vi "Compass Loop.vi"   [LabVIEW 2009]
uses:
  <vilib>/Platform/TimedLoop/XDataNode/XDataNode.xnode
  <vilib>/Platform/TimedLoop/XDataNode/loadlvalarms.vi
  <vilib>/Platform/TimedLoop/XDataNode/timing_clust.ctl
  <vilib>/Platform/TimedLoop/XDataNode/nitl_modes.ctl
  <vilib>/Platform/TimedLoop/XDataNode/wakeup.ctl
  TypeDefs/Sensor TypeDefs/FPGA Main ref.ctl
  <vilib>/userDefined/High Color/nirio_resource_hc.ctl
  <vilib>/rvi/interface/nirviOpenFPGA/nirviOpenFPGA.xnode
  FPGA Bitfiles/Q_IGVC_2010.lvproj_FPGA Target_FPGA_MAIN.vi.lvbitx
  <vilib>/FPGAPlugInAG/cRIO-9113/nirviIntfOpen_cRIO-9113.vi
  Functional Global Variables/Actions for FG's.ctl
  UI Comm/Watchdog Dish Labels.ctl
  <vilib>/Platform/TimedLoop/XDataNode/XDNodeRunTimeDep.lvlib
types:
  T1 = typedef "XDNodeRunTimeDep.lvlib/timing_clust.ctl" = cluster{"Expected End [f-1]":u64, "Actual End [f-1]":u64, "Finished Late? [f-1]":bool, "Expected End [i-1]":u64, "Actual End [i-1]":u64, "Finished Late? [i-1]":bool, "Expected Start [i]":u64, "Actual Start [i]":u64, "Expected Start [f]":u64, "Actual Start [f]":u64, "Source Name":string, "Structure Name":string, "Period":i64, "Deadline":i64, "Offset":i64, "Start":i64, "Priority":i32, "Timeout":i32, "Mode":T2, "Wakeup Reason":T3, "Error":errorcluster, "Source Type":string, "Secondary Source Type":string, "Global End Time":u64, "Global Start Time":u64, "Frame Duration":u64, "Iteration Duration":u64, "Assigned CPU":i32, "I/O Scan Engine Mode":u32}
  T2 = typedef "XDNodeRunTimeDep.lvlib/nitl_modes.ctl" = enum32{"No Change", "Process missed periods, maintain original phase", "Discard missed periods, maintain original phase", "Process missed periods, ignore original phase", "Discard missed periods, ignore original phase"}
  T3 = typedef "XDNodeRunTimeDep.lvlib/wakeup.ctl" = enum32{"Normal", "Aborted", "Asynchronous wakeup", "Timing source error", "Timed loop error", "Timeout"}
  T4 = typedef "FPGA Main ref.ctl" = refnum<k20>
  T5 = typedef "nirio_resource_hc.ctl" = tag
  T6 = cluster{"signature":u8[], "vi signatures match":bool, "signature register address":u32, "reset register address":u32, "control register address":u32, "interrupt base address":u32, "Bitstream Version":u32, "DMA Configuration":cluster{"Name":string, "Depth":u32, "Write? (Deprecated:Use Implementation)":bool, "Physical Channel":u32, "Base Address":u32, "Data Width":u32, "Data Type":enum32{"Boolean", "I8", "I16", "I32", "I64", "U8", "U16", "U32", "U64", "FXP"}, "FXP Properties":variant, "Write Window Address":u32, "Implementation":enum16{"niFpgaTargetToHost", "niFpgaHostToTarget", "niFpgaPeerToPeerWriter", "niFpgaPeerToPeerReader", "niCoreTargetToHost", "niCoreHostToTarget"}, "Control Set":u32}[], "run when loaded?":bool, "reset register size in bits":u32, "compilation results xml":string}
  T7 = typedef "Actions for FG's.ctl" = enum16{"Read", "Write"}
  T8 = typedef "Watchdog Dish Labels.ctl" = enum16{"GPS", "SICK", "Compass", "Cameras", "Motor Controller", "Debug", "RC Receiver"}
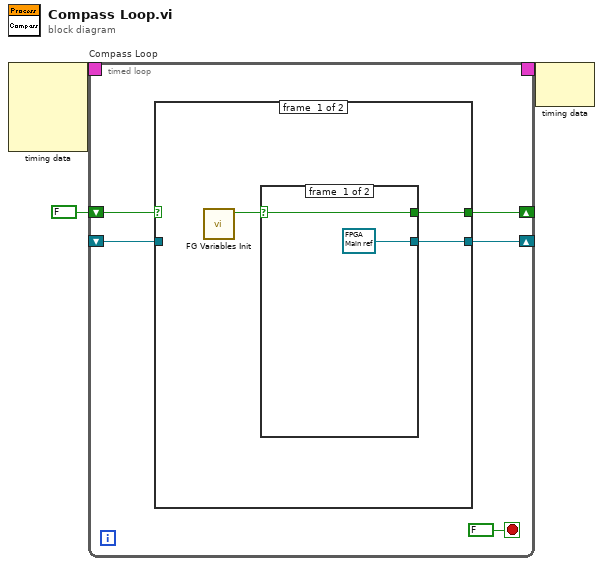
[diagram p0: block diagram]
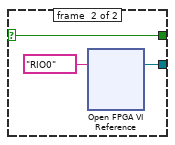
[diagram p2: hidden frame]
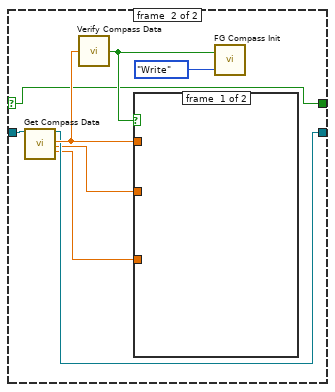
[diagram p3: hidden frame]
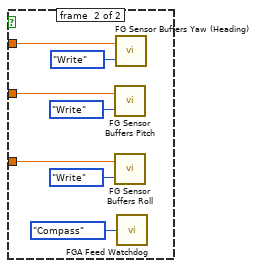
[diagram p4: hidden frame]
diagram:
  n1 = node-c288() -> (w3:T1)  [unwired: 4 in]
  n2 = timed-loop "Compass Loop" {
    timing: w3 -> [_]
    timing-out: [_] -> w2
    shift-right: [w6] -> _
    shift-left: _ -> [w7]
    shift-right: [w4] -> _
    shift-left: FALSE -> [w5]
    stop <- FALSE stop-if-true
    n3 = case shown="False" w5 {
      selector: w5 -> [_ w31]
      tunnel: w7 -> [_ w34]
      tunnel: [w10 w30] -> w6
      tunnel: [w9 w31] -> w4
      frame #0 {
        n4 = call "FG Variables Init.vi"() -> ("Variables Init out"=w11:bool)  [unwired: 11 in]
        n5 = case shown="True" w11 {
          selector: w11 -> [w13 w16]
          tunnel: [w13 w16] -> w9
          tunnel: [T4 refnum ("FPGA VI Reference out") w14] -> w10
          frame #0 {
          }
          frame #1 {
            n6 = xnode "Open FPGA VI Reference"("resource name"=T5 "RIO0") -> ("FPGA VI Reference Out"=w14:refnum<k20>)  [unwired: 1 in, 1 out]
          }
        }
      }
      frame #1 {
        n7 = call "Get Compass Data.vi"("FPGA_MAIN ref in"=w34) -> ("FPGA_MAIN ref out"=w30:T4, "Compass Bearing"=w32:dbl, "Pitch"=w29:dbl, "Roll"=w28:dbl)  [unwired: 14 in, 1 out]
        n8 = call "Verify Compass Data.vi"("Compass Data"=w32) -> ("Data OK?"=w33:bool)
        n9 = case shown="True" w33 {
          tunnel: w32 -> [_ w42]
          tunnel: w29 -> [_ w37]
          tunnel: w28 -> [_ w36]
          frame #0 {
          }
          frame #1 {
            n10 = call "FG Sensor Buffers Pitch.vi"("FG Action (Read)"=Actions_for_FG's."Write", "Pitch Buffer in"=w37) -> ()  [unwired: 1 in, 1 out]
            n11 = call "FG Sensor Buffers Roll.vi"("FG Action (Read)"=Actions_for_FG's."Write", "Roll Buffer in"=w36) -> ()  [unwired: 1 in, 1 out]
            n12 = call "FG Sensor Buffers Yaw (Heading).vi"("FG Action (Read)"=Actions_for_FG's."Write", "Yaw Buffer In"=w42) -> ()  [unwired: 1 in, 1 out]
            n13 = call "FGA Feed Watchdog.vi"("Watchdog Dish"=Watchdog_Dish_Labels."Compass") -> ()  [unwired: 1 out]
          }
        }
        n14 = call "FG Compass Init.vi"("FG Action"=Actions_for_FG's."Write", "Compass Init in"=w33) -> ()  [unwired: 1 out]
      }
    }
  }
  n15 = node-c288(w2) -> ()  [unwired: 1 out]
